vi "Default File Path.vi"(8 "error in (no error)":errorcluster) -> (0 "error out":errorcluster, 3 "Default File Path":path)   [LabVIEW 2020, in "RxnRover.lvlib" / "User Preferences File.lvclass"]
doc: "Gets the default directory to store the user preferences file based on the current operating system. The operating system name is read from OS.Name on a Application property node."
uses:
  User Preferences File.lvclass
  <vilib>/Utility/config.llb/Read Key (Path).vi
  <vilib>/Utility/config.llb/NI_LVConfig.lvlib
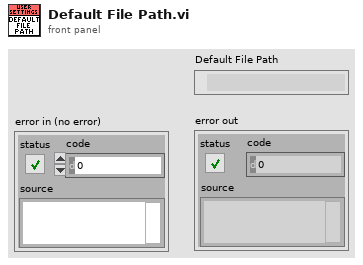
[diagram p1: front panel]
types:
  T1 = typedef "NI_LVConfig.lvlib/Config Data RefNum.ctl" = refnum<k1>
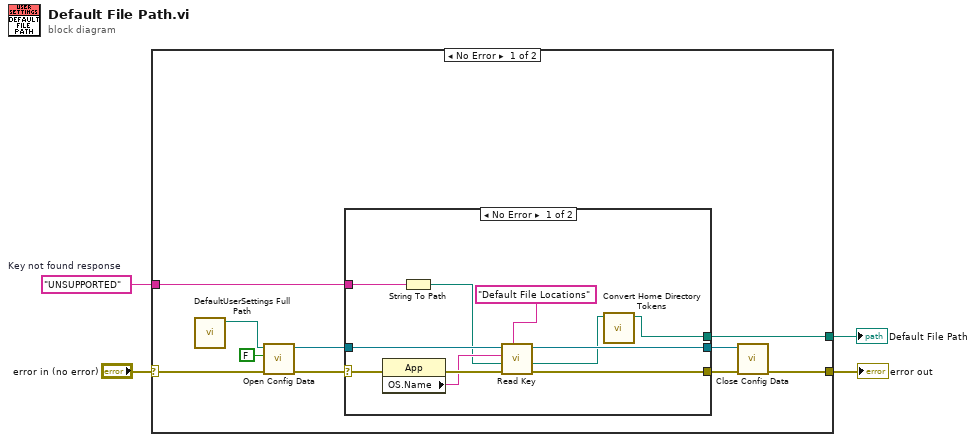
[diagram p0: block diagram]
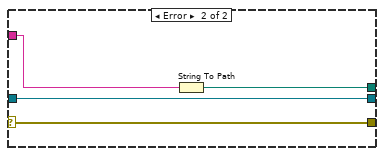
[diagram p2: hidden frame]
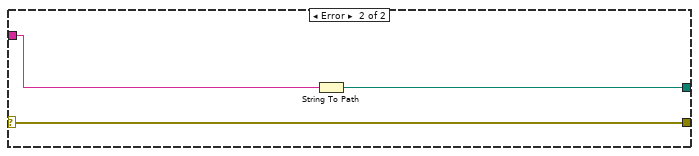
[diagram p3: hidden frame]
diagram:
  w1 = "UNSUPPORTED"  # Key not found response
  n1 = case shown="No Error" "error in (no error)" {
    selector: "error in (no error)" -> [w14 w32]
    tunnel: [w10 w32] -> w3
    tunnel: [w9 w30] -> w2
    tunnel: w1 -> [w8 w31]
    frame No Error {
      n2 = call "DefaultUserSettings Full Path.vi"() -> ("DefaultUserSettings Full Path"=w6:path)  [unwired: 11 in]
      n3 = call <vilib>:"Open Config Data.vi"("error in (no error)"=w14, "create file if necessary (T)"=FALSE, "configuration file path"=w6) -> ("error out"=w5:errorcluster, "refnum"=w13:T1)  [unwired: 6 in, 1 out]
      n4 = case shown="No Error" w5 {
        selector: w5 -> [w18 w29]
        tunnel: w13 -> [w25 w28]
        tunnel: [w21 w29] -> w12
        tunnel: [w20 w28] -> w11
        tunnel: [w15 w26] -> w9
        tunnel: w8 -> [w19 w27]
        frame No Error {
          n5 = property class="App"(error in=w18) -> (error out=w24:errorcluster, "OS.Name"=w23:string)  [unwired: 1 in, 1 out]
          n6 = String To Path(string=w19) -> (path=w17:path)
          n7 = call-poly <vilib>:"Read Key.vi"("section"="Default File Locations", "error in (no error)"=w24, "default value"=w17, "key"=w23, "refnum"=w25) -> ("error out"=w21:errorcluster, "value"=w16:path, "refnum out"=w20:T1)  [unwired: 3 in, 1 out]
          n8 = call "Convert Home Directory Tokens.vi"("Home Directory Token"=w16) -> ("Home Directory"=w15:path)  [unwired: 10 in]
        }
        frame Error {
          n9 = String To Path(string=w27) -> (path=w26:path)
        }
      }
      n10 = call <vilib>:"Close Config Data.vi"("error in (no error)"=w12, "refnum"=w11) -> ("error out"=w10:errorcluster)  [unwired: 8 in, 1 out]
    }
    frame Error {
      n11 = String To Path(string=w31) -> (path=w30:path)
    }
  }
  "error out" <- w3
  "Default File Path" <- w2
